vi "2 LED Serial Sequence With Jump.vi"(6 "Jump Tag Name":string="Boolean processing result 0", 8 "Tag Name 2":string="Boolean processing result 0", 9 "Tag Name 1":string="Boolean processing result 0", 10 "Name":string="Led Sequence") -> (2 "Sequence out":refnum<class "Sequence Config.lvclass">)   [LabVIEW 2015, in "Sequencer Module tests.lvlib"]
uses:
  Sequencer Module tests.lvlib
  classes/Sequence/Config/Sequence Config.lvclass
  basic steps/Wait Step/Config/Wait Step Config.lvclass
  basic steps/Update Tag Step/Config/Update Tag Configuration/Update Tag Config.lvclass
  <vilib>/NI/Tag Bus Module Framework/channel/channel classification.ctl
  <vilib>/NI/Tag Bus/tag/Data Type.ctl
  basic steps/Conditional Jump Step/Config/Conditional Jump Step Config.lvclass
  <vilib>/NI/Tag Bus/tag/tag descriptor.lvclass
  <vilib>/NI/Tag Bus Module Framework/channel/TBM channel.lvclass
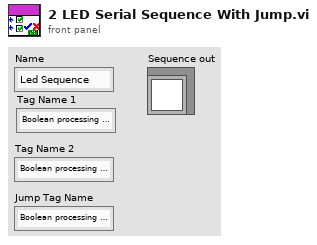
[diagram p1: front panel]
types:
  T1 = typedef "TBM channel.lvclass/channel classification.ctl" = enum16{"input data", "output data", "processing parameter", "processing result"}
  T2 = typedef "tag bus.lvlib/tag descriptor.lvclass/Data Type.ctl" = enum16{"Double", "Single", "I64", "I32", "I16", "I8", "U64", "U32", "U16", "U8", "Boolean", "String", "Array of Double", "Array of Single", "Array of I64", "Array of I32", "Array of I16", "Array of I8", "Array of U64", "Array of U32", "Array of U16", "Array of U8", "Array of Boolean", "Array of String"}
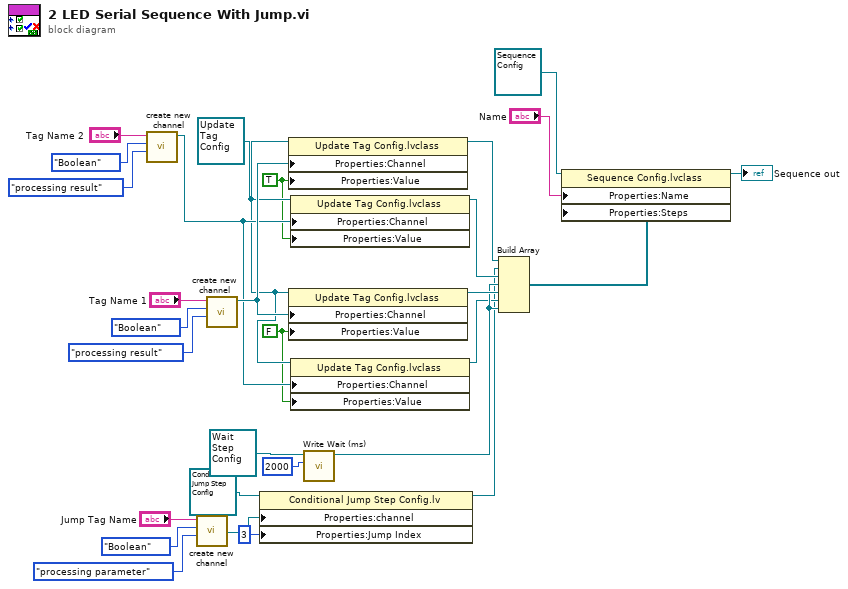
[diagram p0: block diagram]
diagram:
  w12 = FALSE
  w13 = TRUE
  w14 = refnum<class "Update Tag Config.lvclass"> refnum ("Update Tag Config.lvclass")
  n1 = call <vilib>:"create new channel.vi"("channel classification"=channel_classification."processing result", "data type"=Data_Type."Boolean" ("Data Type"), "channel name"="Tag Name 2") -> ("channel"=w15:refnum<class "TBM channel.lvclass">)  [unwired: 8 in]
  n2 = call <vilib>:"create new channel.vi"("channel classification"=channel_classification."processing parameter", "data type"=Data_Type."Boolean" ("Data Type"), "channel name"="Jump Tag Name") -> ("channel"=w4:refnum<class "TBM channel.lvclass">)  [unwired: 8 in]
  n3 = call <vilib>:"create new channel.vi"("channel classification"=channel_classification."processing result", "data type"=Data_Type."Boolean" ("Data Type"), "channel name"="Tag Name 1") -> ("channel"=w19:refnum<class "TBM channel.lvclass">)  [unwired: 8 in]
  n4 = property class="Conditional Jump Step Config.lv"(reference=refnum<class "Conditional Jump Step Config.lvclass"> refnum ("Conditional Jump Step Config.lvclass"), "Properties:channel"=w4, "Properties:Jump Index"=3 ("Jump Index")) -> (reference out=w2:refnum<class "Conditional Jump Step Config.lvclass">)  [unwired: 1 in, 1 out]
  n5 = property class="Update Tag Config.lvclass"(reference=w14, "Properties:Channel"=w19, "Properties:Value"=w13) -> (reference out=w3:refnum<class "Update Tag Config.lvclass">)  [unwired: 1 in, 1 out]
  n6 = property class="Update Tag Config.lvclass"(reference=w14, "Properties:Channel"=w19, "Properties:Value"=w12) -> (reference out=w29:refnum<class "Update Tag Config.lvclass">)  [unwired: 1 in, 1 out]
  n7 = property class="Update Tag Config.lvclass"(reference=w14, "Properties:Channel"=w15, "Properties:Value"=w13) -> (reference out=w11:refnum<class "Update Tag Config.lvclass">)  [unwired: 1 in, 1 out]
  n8 = property class="Update Tag Config.lvclass"(reference=w14, "Properties:Channel"=w15, "Properties:Value"=w12) -> (reference out=w9:refnum<class "Update Tag Config.lvclass">)  [unwired: 1 in, 1 out]
  n9 = call-dynamic "Write Wait (ms).vi"("Wait (ms)"=u32 2000, "Wait Step in"=refnum<class "Wait Step Config.lvclass"> refnum ("Wait Step Config.lvclass")) -> ("Wait Step out"=w10:refnum<class "Wait Step Config.lvclass">)  [unwired: 8 in, 1 out]
  n10 = Build Array(w3, w2, w11, w10, w29, w9, w10) -> (w28:refnum<class "Step Config.lvclass">[])
  n11 = property class="Sequence Config.lvclass"(reference=refnum<class "Sequence Config.lvclass"> refnum ("Sequence Config.lvclass"), "Properties:Name"="Name", "Properties:Steps"=w28) -> (reference out=→"Sequence out":refnum<class "Sequence Config.lvclass">)  [unwired: 1 in, 1 out]
